vi "Set Module Launch Config.vi"() -> (3 "Modules to Launch":T1[](array[typedef]))   [LabVIEW 2021, in "launcher.lvclass"]
uses:
  launcher.lvclass
  <userlib>/S2 Labs/Module Framework/Modules/Base/Launch Module Typdef.ctl
  <userlib>/S2 Labs/Module Framework/Modules/Base/Launch Module Parms.ctl
  bf68eb4f-7c16-44a8-9770-ba0288ee921e.vi
  320ad89a-49d3-4cf8-b10f-d11af02d28f4.vi
  27ef31b6-11a2-42b8-8aae-55a6209030bf.vi
  d70af4c9-52f8-4dab-9035-f98d360ec6a1.vi
  79cffc38-286b-4e18-9dba-9fc99d48f85d.vi
  fba78c4d-d3aa-4513-8d43-73fe61a58e09.vi
  a17c1d87-b89f-4333-86f0-f12587b5e296.vi
  cb943742-f993-4813-8fdb-066abfb48b2a.vi
  258318a4-898c-494c-8f17-c80f93c39a60.vi
  ffadd49c-a3bb-4e6e-bbf8-01701f3eca6b.vi
  aa79f171-7146-4ecf-8844-5aaf61c394f2.vi
  5bfef05e-734f-4853-822d-e9dc9007cb5b.vi
  9b2e93b4-53cc-4b5d-8e97-39068ec62e9b.vi
  d28f6a4e-8195-4828-bc27-6585f4bbc24f.vi
  80072e40-86bc-47ef-8385-6fab86405e22.vi
  <vilib>/JDP Science/JSONtext/Variant to JSON Text.vi
  <vilib>/JDP Science/JSONtext/LVClass Serializer/JSONtext LVClass Serializer.lvclass
  <userlib>/S2 Labs/Module Framework/Modules/Base/Module.lvclass
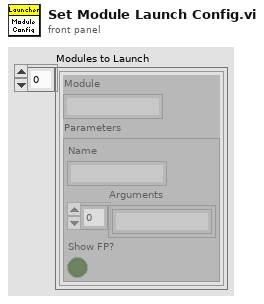
[diagram p1: front panel]
types:
  T1 = typedef "Module.lvclass/Launch Module Typdef.ctl" = cluster{"Module":string, "Parameters":T2}
  T2 = typedef "Module.lvclass/Launch Module Parms.ctl" = cluster{"Name":string, "Arguments":string[], "Show FP?":bool}
  T3 = cluster{"IP Address":string, "Port (502)":u16, "Alias":string[]}
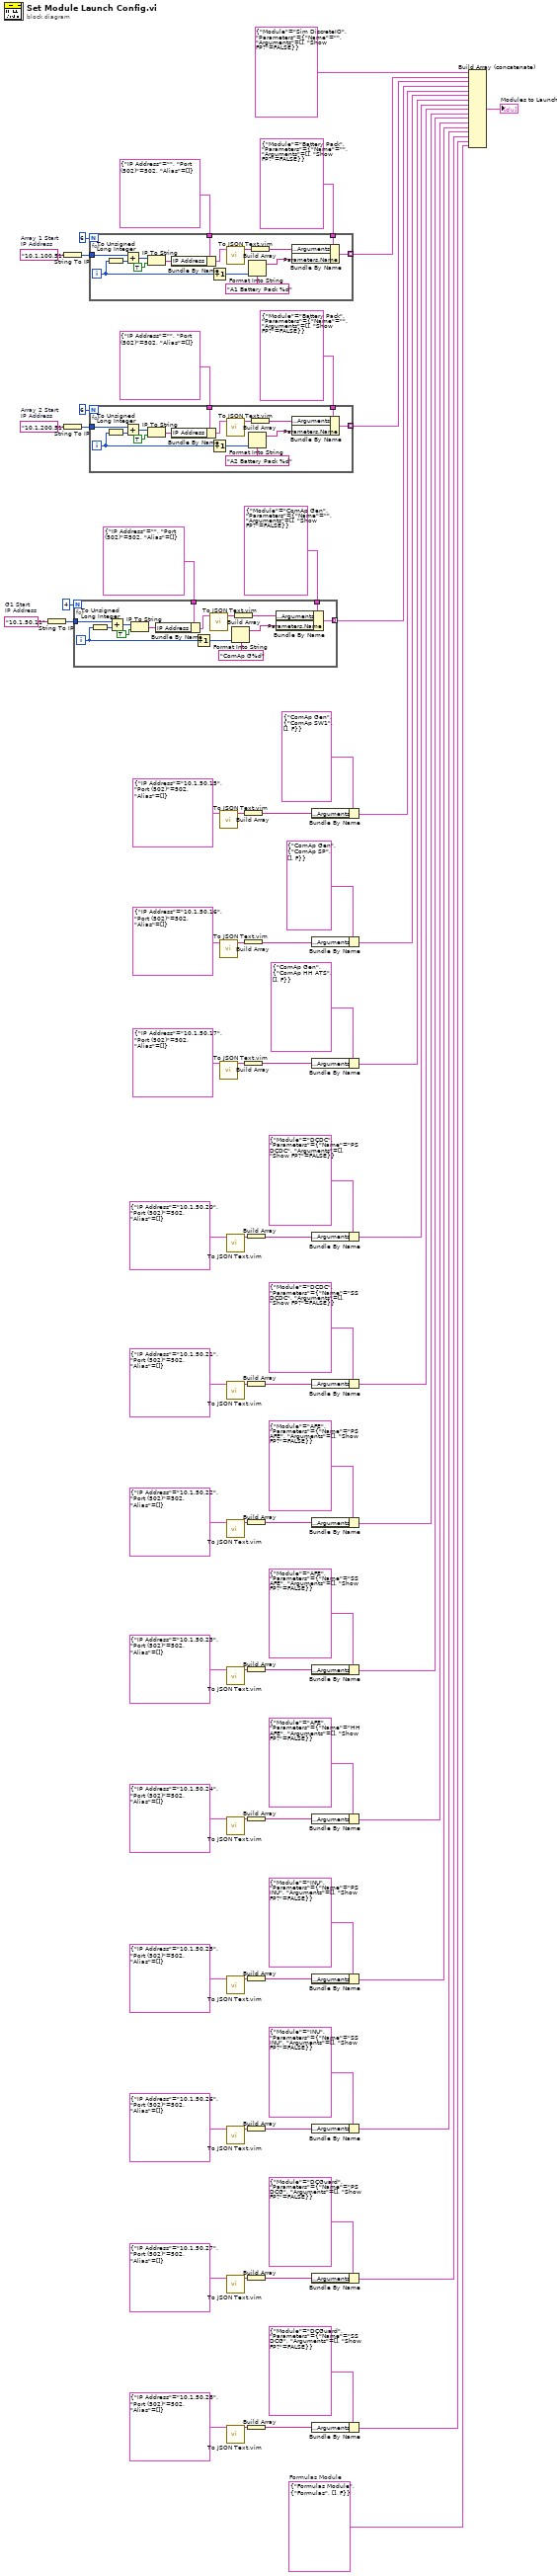
[diagram p0: block diagram]
diagram:
  w21 = "10.1.50.11"  # G1 Start IP Address
  w78 = "10.1.200.51"  # Array 2 Start IP Address
  w75 = "10.1.100.51"  # Array 1 Start IP Address
  w27 = T1 {"Module"="Formulas Module", "Parameters"={"Name"="Formulas", "Arguments"=[], "Show FP?"=FALSE}}  # Formulas Module
  n1 = String To IP(1:w21) -> (0:w20:u32)
  n2 = String To IP(1:w75) -> (0:w76:u32)
  n3 = String To IP(1:w78) -> (0:w77:u32)
  n4 = for {
    N: 4 -> [_]
    tunnel: T3 {"IP Address"="", "Port (502)"=502, "Alias"=[]} -> [w95]
    tunnel: T1 {"Module"="ComAp Gen", "Parameters"={"Name"="", "Arguments"=[], "Show FP?"=FALSE}} ("Launch Module") -> [w93]
    tunnel: [w88] -> w5 mode=indexing
    tunnel: w20 -> [w87]
    i -> [w86]
    n5 = To Unsigned Long Integer(number=w86) -> (unsigned 32bit integer=w85:u32)
    n6 = Add(x=w87, y=w85) -> (x+y=w83:u32)
    n7 = IP To String(1:TRUE ("dot notation? (F)"), 2:w83) -> (0:w82:string)
    n8 = Bundle By Name(cluster=w95, "IP Address"=w82) -> (w94:T3)
    n9 = Increment(x=w86) -> (x+1=w91:i32)
    n10 = call "To JSON Text.vim"("Anything"=w94) -> ("<JSON>"=w96:string)  [unwired: 9 in, 1 out]
    n11 = Format Into String(format string="ComAp G%d", w91) -> (resulting string=w89:string)  [unwired: 2 in, 1 out]
    n12 = Build Array(w96) -> (w92:string[])
    n13 = Bundle By Name(cluster=w93, "Parameters.Arguments"=w92, "Parameters.Name"=w89) -> (w88:T1)
  }
  n14 = for {
    N: 6 -> [_]
    tunnel: T3 {"IP Address"="", "Port (502)"=502, "Alias"=[]} -> [w110]
    tunnel: T1 {"Module"="Battery Pack", "Parameters"={"Name"="", "Arguments"=[], "Show FP?"=FALSE}} ("Launch Module") -> [w108]
    tunnel: [w103] -> w7 mode=indexing
    tunnel: w76 -> [w102]
    i -> [w101]
    n15 = To Unsigned Long Integer(number=w101) -> (unsigned 32bit integer=w100:u32)
    n16 = Add(x=w102, y=w100) -> (x+y=w98:u32)
    n17 = IP To String(1:TRUE ("dot notation? (F)"), 2:w98) -> (0:w97:string)
    n18 = Bundle By Name(cluster=w110, "IP Address"=w97) -> (w109:T3)
    n19 = Increment(x=w101) -> (x+1=w106:i32)
    n20 = call "To JSON Text.vim"("Anything"=w109) -> ("<JSON>"=w111:string)  [unwired: 9 in, 1 out]
    n21 = Format Into String(format string="A1 Battery Pack %d", w106) -> (resulting string=w104:string)  [unwired: 2 in, 1 out]
    n22 = Build Array(w111) -> (w107:string[])
    n23 = Bundle By Name(cluster=w108, "Parameters.Arguments"=w107, "Parameters.Name"=w104) -> (w103:T1)
  }
  n24 = for {
    N: 6 -> [_]
    tunnel: T3 {"IP Address"="", "Port (502)"=502, "Alias"=[]} -> [w125]
    tunnel: T1 {"Module"="Battery Pack", "Parameters"={"Name"="", "Arguments"=[], "Show FP?"=FALSE}} ("Launch Module") -> [w123]
    tunnel: [w118] -> w6 mode=indexing
    tunnel: w77 -> [w117]
    i -> [w116]
    n25 = To Unsigned Long Integer(number=w116) -> (unsigned 32bit integer=w115:u32)
    n26 = Add(x=w117, y=w115) -> (x+y=w113:u32)
    n27 = IP To String(1:TRUE ("dot notation? (F)"), 2:w113) -> (0:w112:string)
    n28 = Bundle By Name(cluster=w125, "IP Address"=w112) -> (w124:T3)
    n29 = Increment(x=w116) -> (x+1=w121:i32)
    n30 = call "To JSON Text.vim"("Anything"=w124) -> ("<JSON>"=w126:string)  [unwired: 9 in, 1 out]
    n31 = Format Into String(format string="A2 Battery Pack %d", w121) -> (resulting string=w119:string)  [unwired: 2 in, 1 out]
    n32 = Build Array(w126) -> (w122:string[])
    n33 = Bundle By Name(cluster=w123, "Parameters.Arguments"=w122, "Parameters.Name"=w119) -> (w118:T1)
  }
  n34 = call "To JSON Text.vim"("Anything"=T3 {"IP Address"="10.1.50.15", "Port (502)"=502, "Alias"=[]}) -> ("<JSON>"=w10:string)  [unwired: 9 in, 1 out]
  n35 = call "To JSON Text.vim"("Anything"=T3 {"IP Address"="10.1.50.16", "Port (502)"=502, "Alias"=[]}) -> ("<JSON>"=w13:string)  [unwired: 9 in, 1 out]
  n36 = call "To JSON Text.vim"("Anything"=T3 {"IP Address"="10.1.50.17", "Port (502)"=502, "Alias"=[]}) -> ("<JSON>"=w18:string)  [unwired: 9 in, 1 out]
  n37 = call "To JSON Text.vim"("Anything"=T3 {"IP Address"="10.1.50.20", "Port (502)"=502, "Alias"=[]}) -> ("<JSON>"=w52:string)  [unwired: 9 in, 1 out]
  n38 = call "To JSON Text.vim"("Anything"=T3 {"IP Address"="10.1.50.21", "Port (502)"=502, "Alias"=[]}) -> ("<JSON>"=w57:string)  [unwired: 9 in, 1 out]
  n39 = call "To JSON Text.vim"("Anything"=T3 {"IP Address"="10.1.50.22", "Port (502)"=502, "Alias"=[]}) -> ("<JSON>"=w69:string)  [unwired: 9 in, 1 out]
  n40 = call "To JSON Text.vim"("Anything"=T3 {"IP Address"="10.1.50.23", "Port (502)"=502, "Alias"=[]}) -> ("<JSON>"=w64:string)  [unwired: 9 in, 1 out]
  n41 = call "To JSON Text.vim"("Anything"=T3 {"IP Address"="10.1.50.24", "Port (502)"=502, "Alias"=[]}) -> ("<JSON>"=w61:string)  [unwired: 9 in, 1 out]
  n42 = call "To JSON Text.vim"("Anything"=T3 {"IP Address"="10.1.50.25", "Port (502)"=502, "Alias"=[]}) -> ("<JSON>"=w40:string)  [unwired: 9 in, 1 out]
  n43 = call "To JSON Text.vim"("Anything"=T3 {"IP Address"="10.1.50.26", "Port (502)"=502, "Alias"=[]}) -> ("<JSON>"=w43:string)  [unwired: 9 in, 1 out]
  n44 = call "To JSON Text.vim"("Anything"=T3 {"IP Address"="10.1.50.27", "Port (502)"=502, "Alias"=[]}) -> ("<JSON>"=w33:string)  [unwired: 9 in, 1 out]
  n45 = call "To JSON Text.vim"("Anything"=T3 {"IP Address"="10.1.50.28", "Port (502)"=502, "Alias"=[]}) -> ("<JSON>"=w30:string)  [unwired: 9 in, 1 out]
  n46 = Build Array(w10) -> (w11:string[])
  n47 = Build Array(w13) -> (w12:string[])
  n48 = Build Array(w18) -> (w19:string[])
  n49 = Build Array(w52) -> (w53:string[])
  n50 = Build Array(w57) -> (w56:string[])
  n51 = Build Array(w69) -> (w68:string[])
  n52 = Build Array(w64) -> (w65:string[])
  n53 = Build Array(w61) -> (w60:string[])
  n54 = Build Array(w40) -> (w39:string[])
  n55 = Build Array(w43) -> (w44:string[])
  n56 = Build Array(w33) -> (w34:string[])
  n57 = Build Array(w30) -> (w29:string[])
  n58 = Bundle By Name(cluster=T1 {"Module"="ComAp Gen", "Parameters"={"Name"="ComAp SW1", "Arguments"=[], "Show FP?"=FALSE}} ("Launch Module"), "Parameters.Arguments"=w11) -> (w4:T1)
  n59 = Bundle By Name(cluster=T1 {"Module"="ComAp Gen", "Parameters"={"Name"="ComAp SP", "Arguments"=[], "Show FP?"=FALSE}} ("Launch Module"), "Parameters.Arguments"=w12) -> (w3:T1)
  n60 = Bundle By Name(cluster=T1 {"Module"="ComAp Gen", "Parameters"={"Name"="ComAp HH ATS", "Arguments"=[], "Show FP?"=FALSE}} ("Launch Module"), "Parameters.Arguments"=w19) -> (w2:T1)
  n61 = Bundle By Name(cluster=T1 {"Module"="DCDC", "Parameters"={"Name"="PS DCDC", "Arguments"=[], "Show FP?"=FALSE}} ("Launch Module"), "Parameters.Arguments"=w53) -> (w46:T1)
  n62 = Bundle By Name(cluster=T1 {"Module"="DCDC", "Parameters"={"Name"="SS DCDC", "Arguments"=[], "Show FP?"=FALSE}} ("Launch Module"), "Parameters.Arguments"=w56) -> (w47:T1)
  n63 = Bundle By Name(cluster=T1 {"Module"="AFE", "Parameters"={"Name"="PS AFE", "Arguments"=[], "Show FP?"=FALSE}} ("Launch Module"), "Parameters.Arguments"=w68) -> (w48:T1)
  n64 = Bundle By Name(cluster=T1 {"Module"="AFE", "Parameters"={"Name"="SS AFE", "Arguments"=[], "Show FP?"=FALSE}} ("Launch Module"), "Parameters.Arguments"=w65) -> (w49:T1)
  n65 = Bundle By Name(cluster=T1 {"Module"="AFE", "Parameters"={"Name"="HH AFE", "Arguments"=[], "Show FP?"=FALSE}} ("Launch Module"), "Parameters.Arguments"=w60) -> (w50:T1)
  n66 = Bundle By Name(cluster=T1 {"Module"="INU", "Parameters"={"Name"="PS INU", "Arguments"=[], "Show FP?"=FALSE}} ("Launch Module"), "Parameters.Arguments"=w39) -> (w37:T1)
  n67 = Bundle By Name(cluster=T1 {"Module"="INU", "Parameters"={"Name"="SS INU", "Arguments"=[], "Show FP?"=FALSE}} ("Launch Module"), "Parameters.Arguments"=w44) -> (w36:T1)
  n68 = Bundle By Name(cluster=T1 {"Module"="DCGuard", "Parameters"={"Name"="PS DCG", "Arguments"=[], "Show FP?"=FALSE}} ("Launch Module"), "Parameters.Arguments"=w34) -> (w26:T1)
  n69 = Bundle By Name(cluster=T1 {"Module"="DCGuard", "Parameters"={"Name"="SS DCG", "Arguments"=[], "Show FP?"=FALSE}} ("Launch Module"), "Parameters.Arguments"=w29) -> (w25:T1)
  n70 = Build Array (concatenate)(T1 {"Module"="Sim DiscreteIO", "Parameters"={"Name"="", "Arguments"=[], "Show FP?"=FALSE}} ("Launch Module"), w7, w6, w5, w4, w3, w2, w46, w47, w48, w49, w50, w37, w36, w26, w25, w27) -> (→"Modules to Launch":T1[])
